vi "GetTimeLeft.vi"(8 "error in (no error)":errorcluster, 11 "MGI_Progress Bar in":refnum<class "Progress Bar.lvclass">) -> (0 "error out":errorcluster, 1 "Show Window?":bool, 2 "Time Left":dbl, 3 "MGI_Progress Bar out":refnum<class "Progress Bar.lvclass">)   [LabVIEW 2016, in "Progress Bar.lvclass"]
doc: "Calculates the time left by keeping track of the average time each step takes and how many steps are left to take.\n\nYou can override this method to use a differnt time left calculation\n\nCopyright: MGI\nAuthored by: Derek Trepanier"
uses:
  <userlib>/_MGI/User Interface/Progress Bar/Progress Bar.lvclass
  <userlib>/_MGI/User Interface/Progress Bar/Progress Bar.lvclass/Progress Bar.ctl
  <userlib>/_MGI/User Interface/Progress Bar/Progress Bar Settings/Progress Bar Settings.lvclass
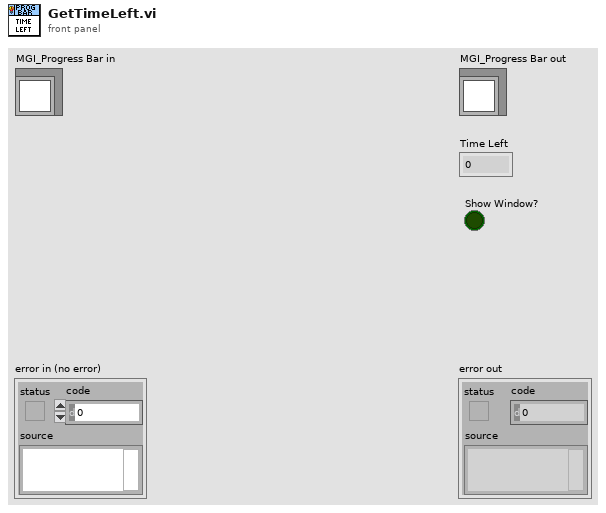
[diagram p1: front panel]
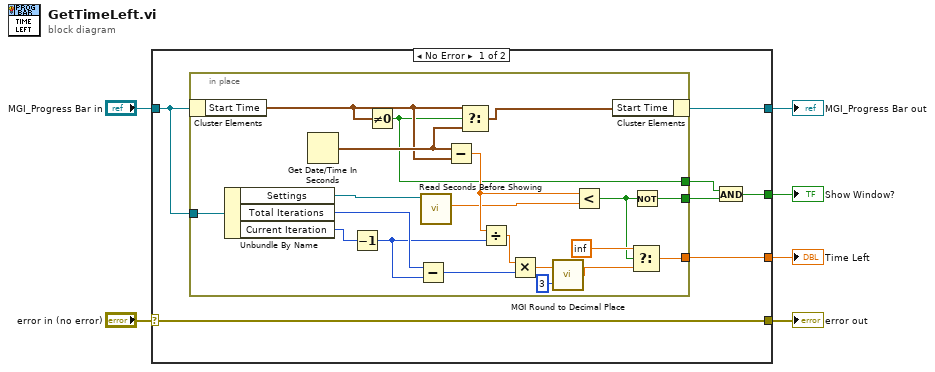
[diagram p0: block diagram]
diagram:
  n1 = case shown="No Error" "error in (no error)" {
    selector: "error in (no error)" -> [w13 w35]
    tunnel: [w13 w35] -> w5
    tunnel: [w12 w34] -> w3
    tunnel: "MGI_Progress Bar in" -> [w11 w34]
    tunnel: [w10 _] -> w2
    tunnel: [w8 _] -> w1
    frame No Error {
      n2 = in-place {
        in-place-border: w11 -> [w32]
        in-place-border: [w24] -> w10
        in-place-border: [w18] -> w9
        in-place-border: [w16] -> w7
        n3 = in-place-cluster #1(w11) -> ("Start Time"=w30:timestamp)
        n4 = Unbundle By Name(w32) -> ("Settings"=w15:refnum<class "Progress Bar Settings.lvclass">, "Total Iterations"=w29:i32, "Current Iteration"=w28:i32)
        n5 = Get Date/Time In Seconds() -> (seconds since 1Jan1904=w31:timestamp)
        n6 = Decrement(x=w28) -> (x-1=w22:i32)
        n7 = Not Equal To 0?(x=w30) -> (x != 0?=w16:bool)
        n8 = Subtract(x=w29, y=w22) -> (x-y=w27:i32)
        n9 = call-dynamic "Read Seconds Before Showing.vi"("MGI_Progress Bar Options in"=w15) -> ("Seconds Before Showing"=w14:dbl)  [unwired: 8 in, 2 out]
        n10 = Subtract(x=w31, y=w30) -> (x-y=w17:dbl)
        n11 = Select(t=w30, s=w16, f=w31) -> (s? t:f=w33:timestamp)
        n12 = Divide(x=w17, y=w22) -> (x/y=w26:dbl)
        n13 = Multiply(x=w26, y=w27) -> (x*y=w25:dbl)
        n14 = call <userlib>:"MGI Round to Decimal Place.vi"("Decimal Digits"=3, "Number"=w25) -> ("Rounded"=w21:dbl)  [unwired: 1 in]
        n15 = Less?(x=w17, y=w14) -> (x < y?=w19:bool)
        n16 = in-place-cluster #1("Start Time"=w33) -> (w12:refnum<class "Progress Bar.lvclass">)
        n17 = Select(t=inf, s=w19, f=w21) -> (s? t:f=w24:dbl)
        n18 = Not(x=w19) -> (.not. x?=w18:bool)
      }
      n19 = And(x=w7, y=w9) -> (x .and. y?=w8:bool)
    }
    frame Error {
    }
  }
  "error out" <- w5
  "MGI_Progress Bar out" <- w3
  "Time Left" <- w2
  "Show Window?" <- w1
